vi "Event Structure Data.vi"() -> ()   [LabVIEW 2017]
uses:
  <vilib>/Analysis/NI_AALBase.lvlib
panel:
  in  "Plot Colour":u32(colorbox)
  in  "Stop":bool
  in  "Amplitude":dbl(knob) scale=0.0..10.0
  out "Waveform Chart":dbl[](graph)
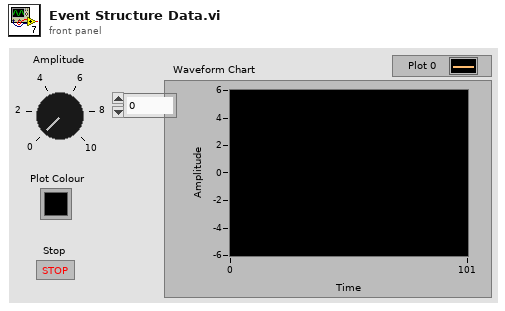
[diagram p1: front panel]
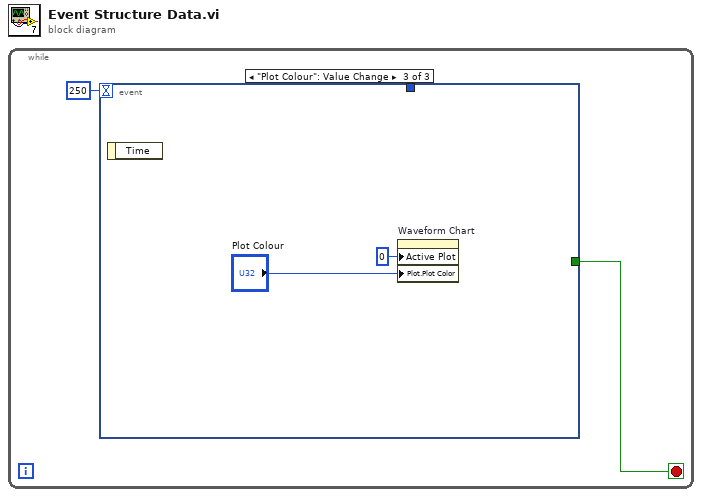
[diagram p0: block diagram]
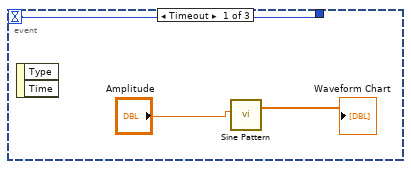
[diagram p2: hidden frame]
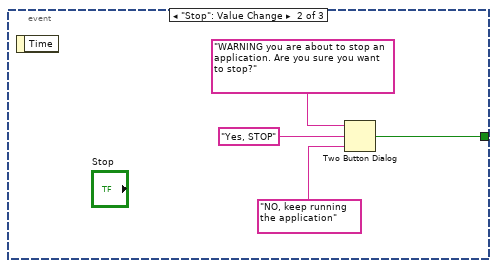
[diagram p3: hidden frame]
diagram:
  n1 = while {
    stop <- w2 stop-if-true
    n2 = event shown="[2] \"Plot Colour\": Value Change" {
      selector: _ -> [_ _ _]
      dyn-events: _ -> [_ _ _]
      timeout: 250 -> [w5 _ _]
      tunnel: [w5 _ _] -> _
      tunnel: [_ w6 _] -> w2
      event Timeout {
        n3 = event-data() -> ()  [unwired: 1 in, 2 out]
        n4 = call <vilib>:"Sine Pattern.vi"("amplitude"="Amplitude") -> ("Sinusoidal Pattern"=→"Waveform Chart":dbl[])  [unwired: 3 in, 1 out]
      }
      event "Stop": Value Change {
        n5 = event-data() -> ()  [unwired: 1 in, 1 out]
        n6 = Two Button Dialog(message="WARNING you are about to stop an application. Are you sure you want to stop?", 1:"NO, keep running the application", 2:"Yes, STOP" ("T button name (\"OK\")")) -> (T button?=w6:bool)
      }
      event "Plot Colour": Value Change {
        n7 = event-data() -> ()  [unwired: 1 in, 1 out]
        n8 = property on="Waveform Chart" class="WFChart (strict)"("Active Plot"=u32 0, "Plot.Plot Color"="Plot Colour") -> ()  [unwired: 2 in, 2 out]
      }
    }
  }
